vi "color_temp_sub_vi.vi"(0 "spectra":dbl[][](array[numeric]) format="%0.3f", 1 "sensesitivity":dbl[][](array[numeric]) format="%0.3f") -> (2 "x":dbl, 3 "y":dbl, 4 "z":dbl)   [LabVIEW 2022 SP3]
uses:
  <vilib>/gmath/NI_Gmath.lvlib
panel:
  out "XY Graph 4":cluster{dbl[], dbl[]}[](graph)
  out "B":dbl
  out "G":dbl
  out "R":dbl
  out "XY Graph 3":cluster{"all rows":dbl[], "all rows":dbl[]}[](graph)
  out "XY Graph 2":cluster{"all rows":dbl[], "all rows":dbl[]}[](graph)
  in  "xyz":dbl[][](array[numeric])=[[380.0, 0.0014, 0.0, 0.0065], [385.0, 0.0022, 0.0001, 0.0105], [390.0, 0.0042, 0.0001, 0.0201], [395.0, 0.0076, 0.0002, 0.0362], [400.0, 0.0143, 0.0004, 0.0679], [405.0, 0.0232, 0.0006, 0.1102], [410.0, 0.0435, 0.0012, 0.2074], [415.0, 0.0776, 0.0022, 0.3713], [420.0, 0.1344, 0.004, 0.6456], [425.0, 0.2148, 0.0073, 1.0391], [430.0, 0.2839, 0.0116, 1.3856], [435.0, 0.3285, 0.0168, 1.623], [440.0, 0.3483, 0.023, 1.7471], [445.0, 0.3481, 0.0298, 1.7826], [450.0, 0.3362, 0.038, 1.7721], [455.0, 0.3187, 0.048, 1.7441], [460.0, 0.2908, 0.06, 1.6692], [465.0, 0.2511, 0.0739, 1.5281], [470.0, 0.1954, 0.091, 1.2876], [475.0, 0.1421, 0.1126, 1.0419], [480.0, 0.0956, 0.139, 0.813], [485.0, 0.058, 0.1693, 0.6162], [490.0, 0.032, 0.208, 0.4652], [495.0, 0.0147, 0.2586, 0.3533], [500.0, 0.0049, 0.323, 0.272], [505.0, 0.0024, 0.4073, 0.2123], [510.0, 0.0093, 0.503, 0.1582], [515.0, 0.0291, 0.6082, 0.1117], [520.0, 0.0633, 0.71, 0.0782], [525.0, 0.1096, 0.7932, 0.0573], [530.0, 0.1655, 0.862, 0.0422], [535.0, 0.2257, 0.9149, 0.0298], [540.0, 0.2904, 0.954, 0.0203], [545.0, 0.3597, 0.9803, 0.0134], [550.0, 0.4334, 0.995, 0.0087], [555.0, 0.5121, 1.0002, 0.0057], [560.0, 0.5945, 0.995, 0.0039], [565.0, 0.6784, 0.9786, 0.0027], [570.0, 0.7621, 0.952, 0.0021], [575.0, 0.8425, 0.9154, 0.0018], [580.0, 0.9163, 0.87, 0.0017], [585.0, 0.9786, 0.8163, 0.0014], [590.0, 1.0263, 0.757, 0.0011], [595.0, 1.0567, 0.6949, 0.001], [600.0, 1.0622, 0.631, 0.0008], [605.0, 1.0456, 0.5668, 0.0006], [610.0, 1.0026, 0.503, 0.0003], [615.0, 0.9384, 0.4412, 0.0002], [620.0, 0.8544, 0.381, 0.0002], [625.0, 0.7514, 0.321, 0.0001], [630.0, 0.6424, 0.265, 0.0], [635.0, 0.5419, 0.217, 0.0], [640.0, 0.4479, 0.175, 0.0], [645.0, 0.3608, 0.1382, 0.0], [650.0, 0.2835, 0.107, 0.0], [655.0, 0.2187, 0.0816, 0.0], [660.0, 0.1649, 0.061, 0.0], [665.0, 0.1212, 0.0446, 0.0], [670.0, 0.0874, 0.032, 0.0], [675.0, 0.0636, 0.0232, 0.0], [680.0, 0.0468, 0.017, 0.0], [685.0, 0.0329, 0.0119, 0.0], [690.0, 0.0227, 0.0082, 0.0], [695.0, 0.0158, 0.0057, 0.0], [700.0, 0.0114, 0.0041, 0.0], [705.0, 0.0081, 0.0029, 0.0], [710.0, 0.0058, 0.0021, 0.0], [715.0, 0.0041, 0.0015, 0.0], [720.0, 0.0029, 0.001, 0.0], [725.0, 0.002, 0.0007, 0.0], [730.0, 0.0014, 0.0005, 0.0], [735.0, 0.001, 0.0004, 0.0], [740.0, 0.0007, 0.0003, 0.0], [745.0, 0.0005, 0.0002, 0.0], [750.0, 0.0003, 0.0001, 0.0], [755.0, 0.0002, 0.0001, 0.0], [760.0, 0.0002, 0.0001, 0.0], [765.0, 0.0001, 0.0, 0.0], [770.0, 0.0001, 0.0, 0.0], [775.0, 0.0, 0.0, 0.0], [780.0, 0.0, 0.0, 0.0]] format="%0.3f"
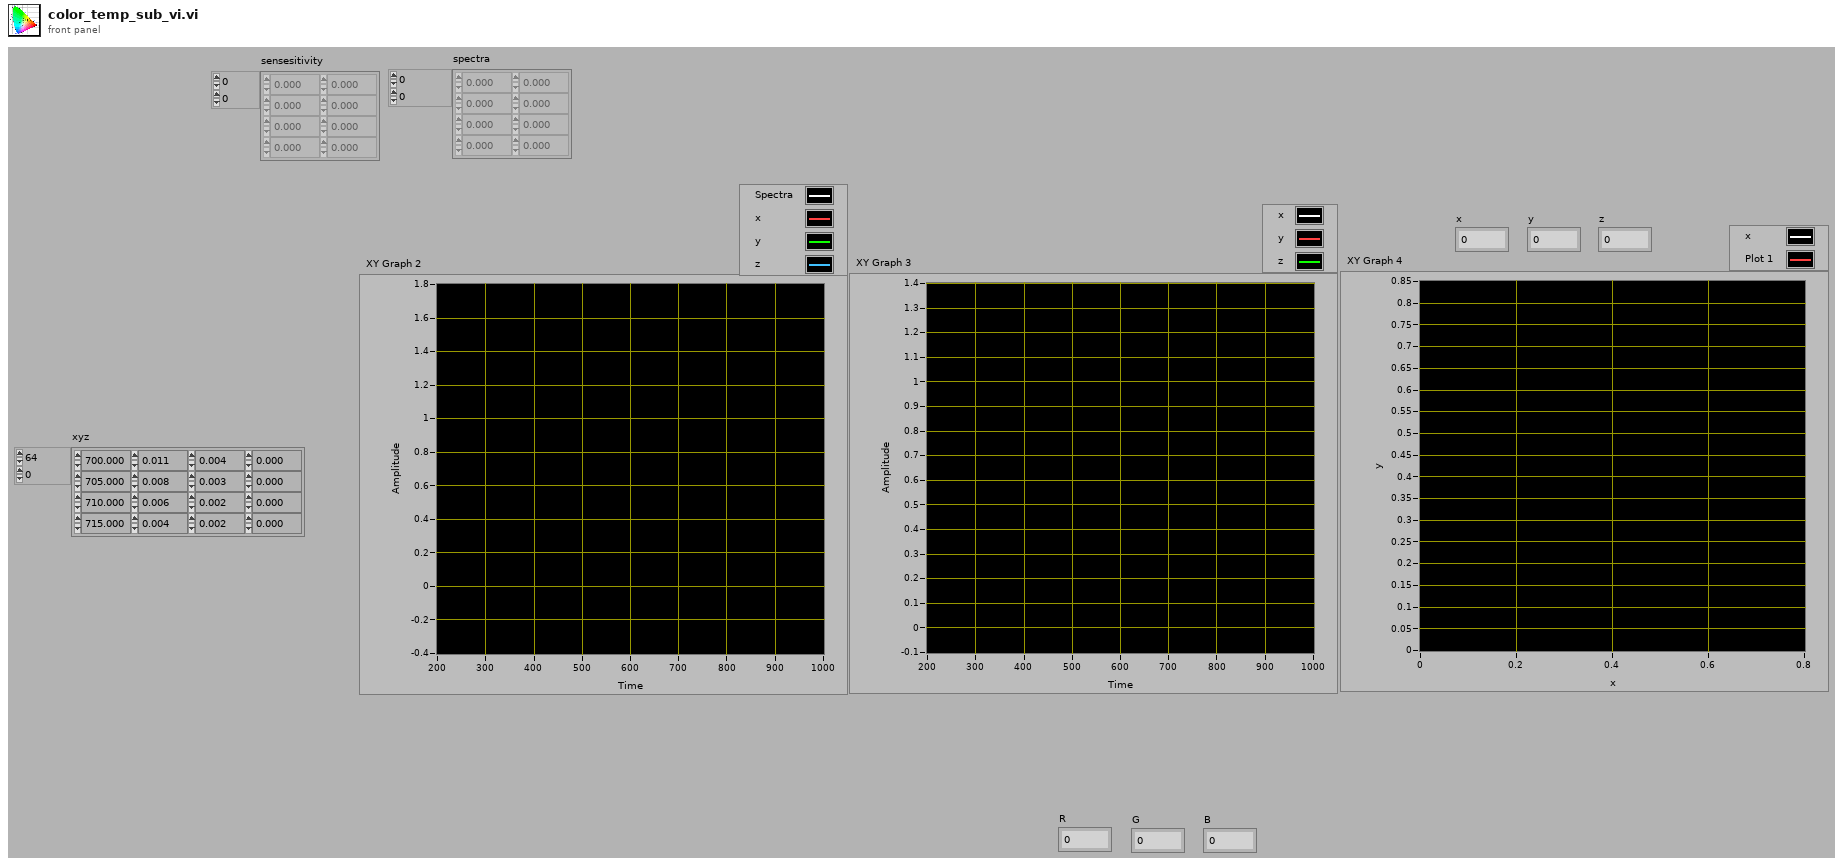
[diagram p1: front panel]
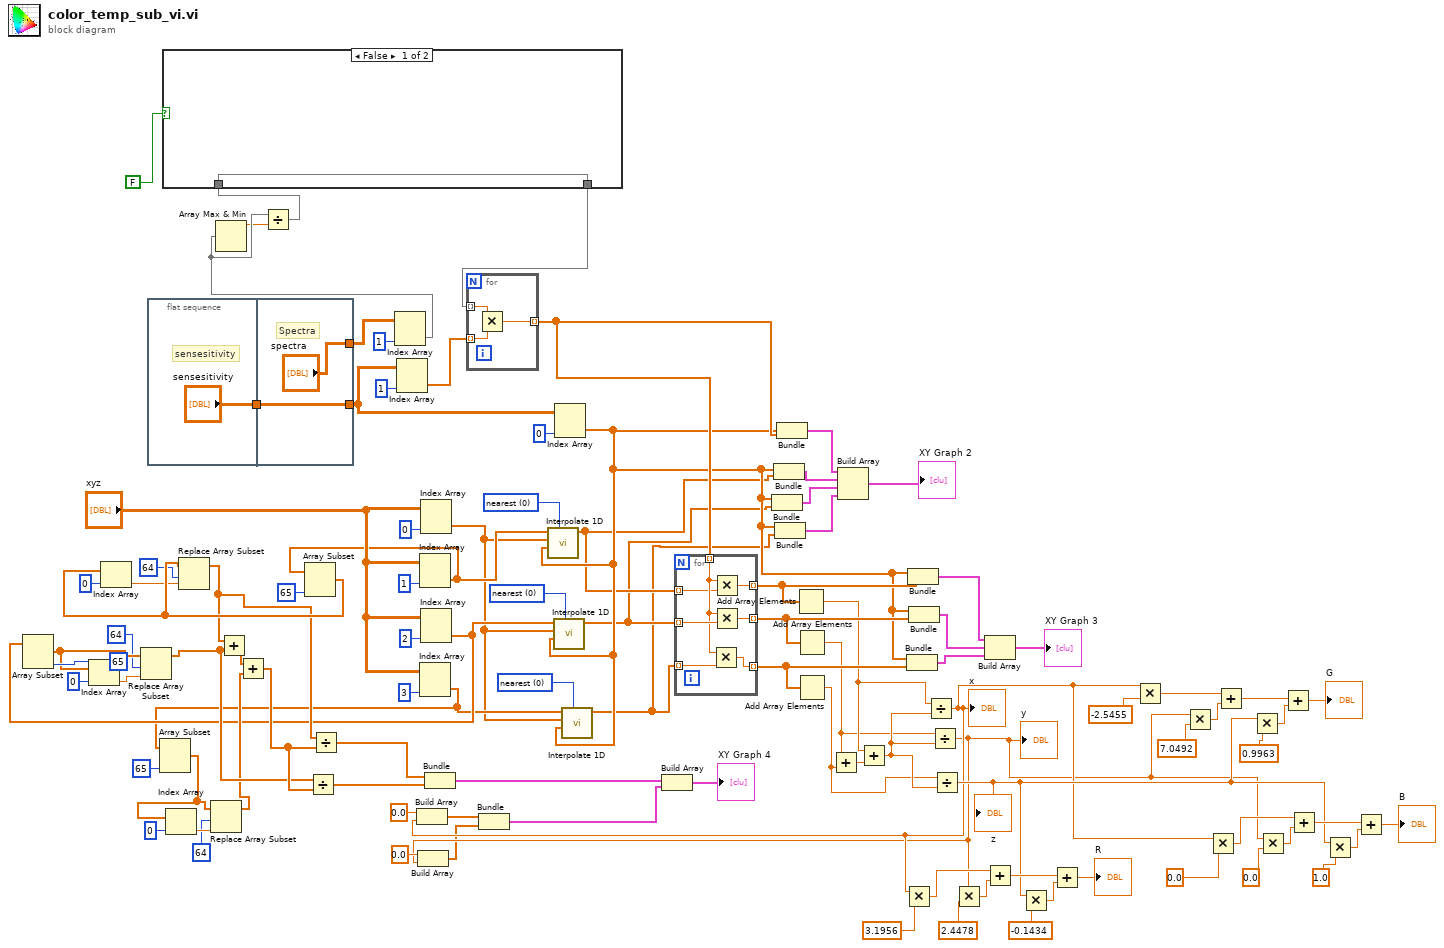
[diagram p0: block diagram]
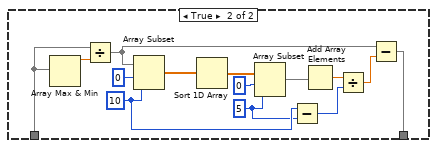
[diagram p2: hidden frame]
diagram:
  w11 = 0 items=["nearest", "linear", "spline", "cubic Hermite", "Lagrange"] ("method")
  w13 = 0 items=["nearest", "linear", "spline", "cubic Hermite", "Lagrange"] ("method")
  w15 = 0 items=["nearest", "linear", "spline", "cubic Hermite", "Lagrange"] ("method")
  n1 = flat-sequence {
    tunnel: ["sensesitivity"] -> w84
    tunnel: [w105] -> w101
    tunnel: w84 -> [w105]
    tunnel: ["spectra"] -> w82
    frame #0 {
      # "sensesitivity"
    }
    frame #1 {
      # "Spectra"
    }
  }
  n2 = Index Array(array=w82, index (col)=1 ("disabled index (col)")) -> (element=w3:dbl[])  [unwired: 1 in]
  n3 = Array Max & Min(array=w3) -> (max value=w2:dbl)  [unwired: 3 out]
  n4 = Divide(x=w3, y=w2) -> (x/y=w1:dbl[])
  n5 = case shown="False" FALSE {
    tunnel: w1 -> [w106 w108]
    tunnel: [w106 w107] -> w80
    frame False {
    }
    frame True {
      w113 = 5 ("length")
      w114 = 10 ("length")
      n6 = Array Max & Min(array=w108) -> (max value=w110:dbl)  [unwired: 3 out]
      n7 = Divide(x=w108, y=w110) -> (x/y=w109:dbl[])
      n8 = Array Subset(array=w109, index=0, length=w114) -> (w119:dbl[])
      n9 = Sort 1D Array(array=w119) -> (sorted array=w118:dbl[])
      n10 = Array Subset(array=w118, index=0, length=w113) -> (w116:dbl[])
      n11 = Subtract(x=w114, y=w113) -> (x-y=w112:i32)
      n12 = Add Array Elements(numeric array=w116) -> (sum=w115:dbl)
      n13 = Divide(x=w115, y=w112) -> (x/y=w111:dbl)
      n14 = Subtract(x=w109, y=w111) -> (x-y=w107:dbl[])
    }
  }
  n15 = Index Array(array=w101, index (col)=1 ("disabled index (col)")) -> (element=w81:dbl[])  [unwired: 1 in]
  n16 = Index Array(array="xyz", index (col)=1 ("disabled index (col)")) -> (element=w14:dbl[])  [unwired: 1 in]
  n17 = Array Subset(array=w14, length=65) -> (w30:dbl[])  [unwired: 1 in]
  n18 = Index Array(array=w30, index=0) -> (element=w29:dbl)
  n19 = Replace Array Subset(array=w30, new element=w29, index=64) -> (w19:dbl[])
  n20 = Index Array(array="xyz", index (col)=3 ("disabled index (col)")) -> (element=w10:dbl[])  [unwired: 1 in]
  n21 = Array Subset(array=w10, length=65) -> (w22:dbl[])  [unwired: 1 in]
  n22 = Index Array(array=w22, index=0) -> (element=w21:dbl)
  n23 = Replace Array Subset(array=w22, new element=w21, index=64) -> (w23:dbl[])
  n24 = Index Array(array="xyz", index (col)=0 ("disabled index (col)")) -> (element=w9:dbl[])  [unwired: 1 in]
  n25 = Index Array(array="xyz", index (col)=2 ("disabled index (col)")) -> (element=w12:dbl[])  [unwired: 1 in]
  n26 = Array Subset(array=w12, length=65) -> (w27:dbl[])  [unwired: 1 in]
  n27 = Index Array(array=w27, index=0) -> (element=w25:dbl)
  n28 = Replace Array Subset(array=w27, new element=w25, index=64) -> (w26:dbl[])
  n29 = Add(x=w19, y=w26) -> (x+y=w49:dbl[])
  n30 = Add(x=w49, y=w23) -> (x+y=w48:dbl[])
  n31 = Divide(x=w26, y=w48) -> (x/y=w46:dbl[])
  n32 = Divide(x=w19, y=w48) -> (x/y=w47:dbl[])
  n33 = Bundle(w47, w46) -> (w45:cluster{dbl[], dbl[]})  [unwired: 1 in]
  n34 = for {
    tunnel: w80 -> [w123] mode=indexing
    tunnel: w81 -> [w122] mode=indexing
    tunnel: [w121] -> w16 mode=indexing
    n35 = Multiply(x=w123, y=w122) -> (x*y=w121:dbl)
  }
  n36 = Index Array(array=w101, index (col)=0 ("disabled index (col)")) -> (element=w7:dbl[])  [unwired: 1 in]
  n37 = call <vilib>:"Interpolate 1D.vi"("method"=w15, "xi"=w7, "X"=w9, "Y"=w14) -> ("yi"=w6:dbl[])  [unwired: 5 in, 2 out]
  n38 = call <vilib>:"Interpolate 1D.vi"("method"=w13, "xi"=w7, "X"=w9, "Y"=w12) -> ("yi"=w5:dbl[])  [unwired: 5 in, 2 out]
  n39 = call <vilib>:"Interpolate 1D.vi"("method"=w11, "xi"=w7, "X"=w9, "Y"=w10) -> ("yi"=w4:dbl[])  [unwired: 5 in, 2 out]
  n40 = for {
    tunnel: w16 -> [w128] mode=indexing
    tunnel: w5 -> [w130] mode=indexing
    tunnel: w4 -> [w129] mode=indexing
    tunnel: [w127] -> w87 mode=indexing
    tunnel: [w126] -> w86 mode=indexing
    tunnel: [w125] -> w85 mode=indexing
    tunnel: w6 -> [w124] mode=indexing
    n41 = Multiply(x=w128, y=w129) -> (x*y=w125:dbl)
    n42 = Multiply(x=w128, y=w124) -> (x*y=w127:dbl)
    n43 = Multiply(x=w128, y=w130) -> (x*y=w126:dbl)
  }
  n44 = Bundle("sensesitivity"=w7, "yi"=w5) -> (w97:cluster{"sensesitivity":dbl[], "yi":dbl[]})  [unwired: 1 in]
  n45 = Bundle("sensesitivity"=w7, "yi"=w6) -> (w98:cluster{"sensesitivity":dbl[], "yi":dbl[]})  [unwired: 1 in]
  n46 = Bundle("sensesitivity"=w7, "yi"=w4) -> (w8:cluster{"sensesitivity":dbl[], "yi":dbl[]})  [unwired: 1 in]
  n47 = Bundle("sensesitivity"=w7, w16) -> (w17:cluster{"sensesitivity":dbl[], dbl[]})  [unwired: 1 in]
  n48 = Add Array Elements(numeric array=w87) -> (sum=w77:dbl)
  n49 = Add Array Elements(numeric array=w86) -> (sum=w76:dbl)
  n50 = Add Array Elements(numeric array=w85) -> (sum=w75:dbl)
  n51 = Add(x=w76, y=w75) -> (x+y=w79:dbl)
  n52 = Build Array(w17, w98, w97, w8) -> (→"XY Graph 2":cluster{"sensesitivity":dbl[], "yi":dbl[]}[])
  n53 = Add(x=w77, y=w79) -> (x+y=w78:dbl)
  n54 = Bundle("sensesitivity"=w7, w85) -> (w89:cluster{"sensesitivity":dbl[], dbl[]})  [unwired: 1 in]
  n55 = Bundle("sensesitivity"=w7, w87) -> (w91:cluster{"sensesitivity":dbl[], dbl[]})  [unwired: 1 in]
  n56 = Bundle("sensesitivity"=w7, w86) -> (w90:cluster{"sensesitivity":dbl[], dbl[]})  [unwired: 1 in]
  n57 = Divide(x=w77, y=w78) -> (x/y=w42:dbl)
  "x" <- w42
  n58 = Build Array(0.0 ("element"), w42) -> (w40:dbl[])
  n59 = Multiply(x=w42, y=3.1956) -> (x*y=w71:dbl)
  n60 = Divide(x=w76, y=w78) -> (x/y=w38:dbl)
  "y" <- w38
  n61 = Build Array(0.0 ("element"), w38) -> (w37:dbl[])
  n62 = Bundle(w40, w37) -> (w44:cluster{dbl[], dbl[]})  [unwired: 1 in]
  n63 = Build Array(w45, w44) -> (→"XY Graph 4":cluster{dbl[], dbl[]}[])
  n64 = Divide(x=w75, y=w78) -> (x/y=w50:dbl)
  "z" <- w50
  n65 = Multiply(x=w38, y=2.4478) -> (x*y=w70:dbl)
  n66 = Build Array(w91, w90, w89) -> (→"XY Graph 3":cluster{"sensesitivity":dbl[], dbl[]}[])
  n67 = Add(x=w71, y=w70) -> (x+y=w68:dbl)
  n68 = Multiply(x=w50, y=-0.1434) -> (x*y=w69:dbl)
  n69 = Add(x=w68, y=w69) -> (x+y=→"R":dbl)
  n70 = Multiply(x=w42, y=-2.5455) -> (x*y=w63:dbl)
  n71 = Multiply(x=w38, y=7.0492) -> (x*y=w62:dbl)
  n72 = Multiply(x=w42, y=0.0) -> (x*y=w55:dbl)
  n73 = Add(x=w63, y=w62) -> (x+y=w60:dbl)
  n74 = Multiply(x=w50, y=0.9963) -> (x*y=w61:dbl)
  n75 = Multiply(x=w38, y=0.0) -> (x*y=w54:dbl)
  n76 = Add(x=w60, y=w61) -> (x+y=→"G":dbl)
  n77 = Add(x=w55, y=w54) -> (x+y=w52:dbl)
  n78 = Multiply(x=w50, y=1.0) -> (x*y=w53:dbl)
  n79 = Add(x=w52, y=w53) -> (x+y=→"B":dbl)
